vi "2.4 Ghz Cutoff UI.vi"() -> ()   [LabVIEW 2010]
uses:
  Drivers/Telemetry/MICS Parameters Global.vi
  Drivers/Telemetry/MICS_ID Global.vi
  Drivers/Telemetry/MICS_Channel Global.vi
panel:
  in  "Number of \"Open Session\" Retry Attempts (3)":i32=3
  in  "400 MHz MICS Power Setting (0x16)":u8=22 format="%02x"
  in  "Attenuation dB (0)":dbl
  in  "MICS inputs":T1={"address"="COM5", "chan"=2, "ID"=4412} {"ID" format="%04x"; "chan" min=1 max=10 step=1}
  in  "2.45 GHz Wakeup Power Array":i8[](array[ring])=[-29, -4, -2, 0, 2, 4, 6, 8, 10, 12, 14, 16, 18, 20] items=["-29"=-29, "-4"=-4, "-2"=-2, "0"=0, "2"=2, "4"=4, "6"=6, "8"=8, "10"=10, "12"=12, "14"=14, "16"=16, "18"=18, "20"=20, ""=22, ""=24, ""=26, ""=27]
  in  "Samples":i32=10
  in  "stop":bool
  out "error out":errorcluster
  out "Percent Success vs. 2.45 GHz Wakeup Power":T2(graph)
  in  "error in (no error)":errorcluster
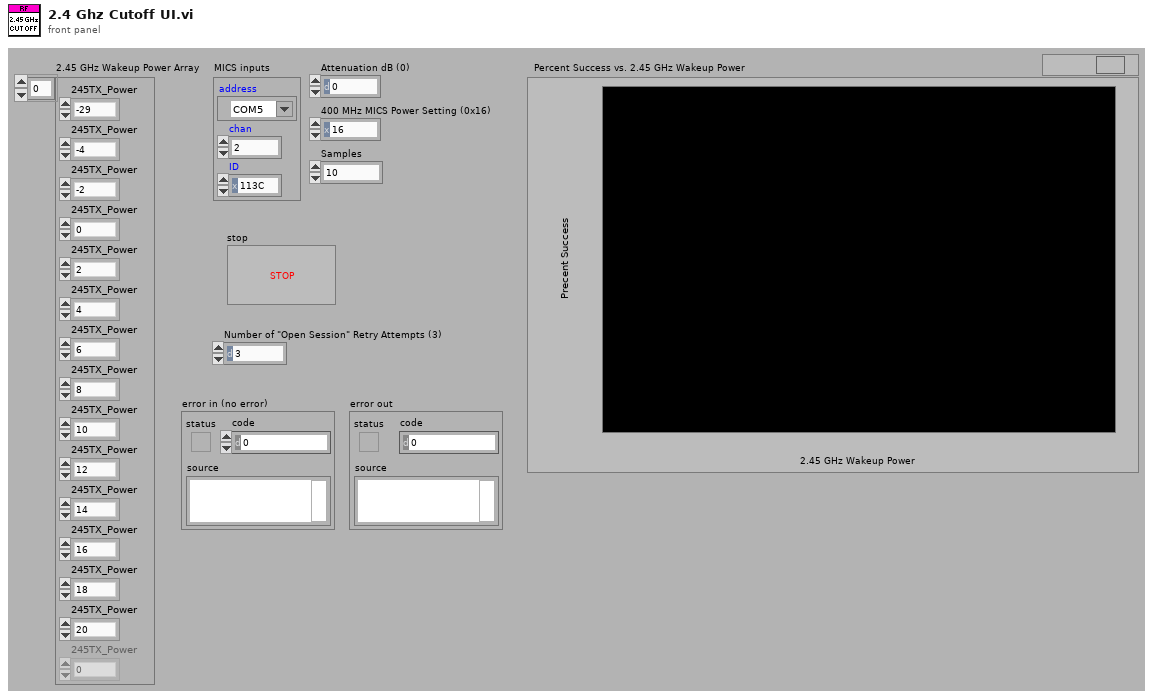
[diagram p1: front panel]
types:
  T1 = cluster{"address":refnum<visa-resource-name>, "chan":u16, "ID":u32}
  T2 = cluster{"245TX_Power":i8, "Percent Successful":dbl}[]
  T3 = cluster{"ConfigFlags":u8, "ImplantID":u32, "CompanyID":u8, "Normal_Comm":cluster{"RF_Channel":u8, "UserData":u8, "TX_Mod":u8, "RX_Mod":u8, "RX_BlockSize":u8, "BlockPerPack":u8, "TX_BlockSize":u8}, "Emerg_Comm":cluster{"RF_Channel":u8, "UserData":u8, "TX_Mod":u8, "RX_Mod":u8, "TX_BlockSize":u8, "BlockPerPack":u8, "RX_BlockSize":u8}, "ImplantRev":u8, "245TX_PowerCal":i8, "245TX_Power":i8, "CCA_RSSI_Thresholds":cluster{"ch0":u16, "ch1":u16, "ch2":u16, "ch3":u16, "ch4":u16, "ch5":u16, "ch6":u16, "ch7":u16, "ch8":u16, "ch9":u16}}
  T4 = cluster{"245TX_Power":i8, "Percent Successful":dbl}
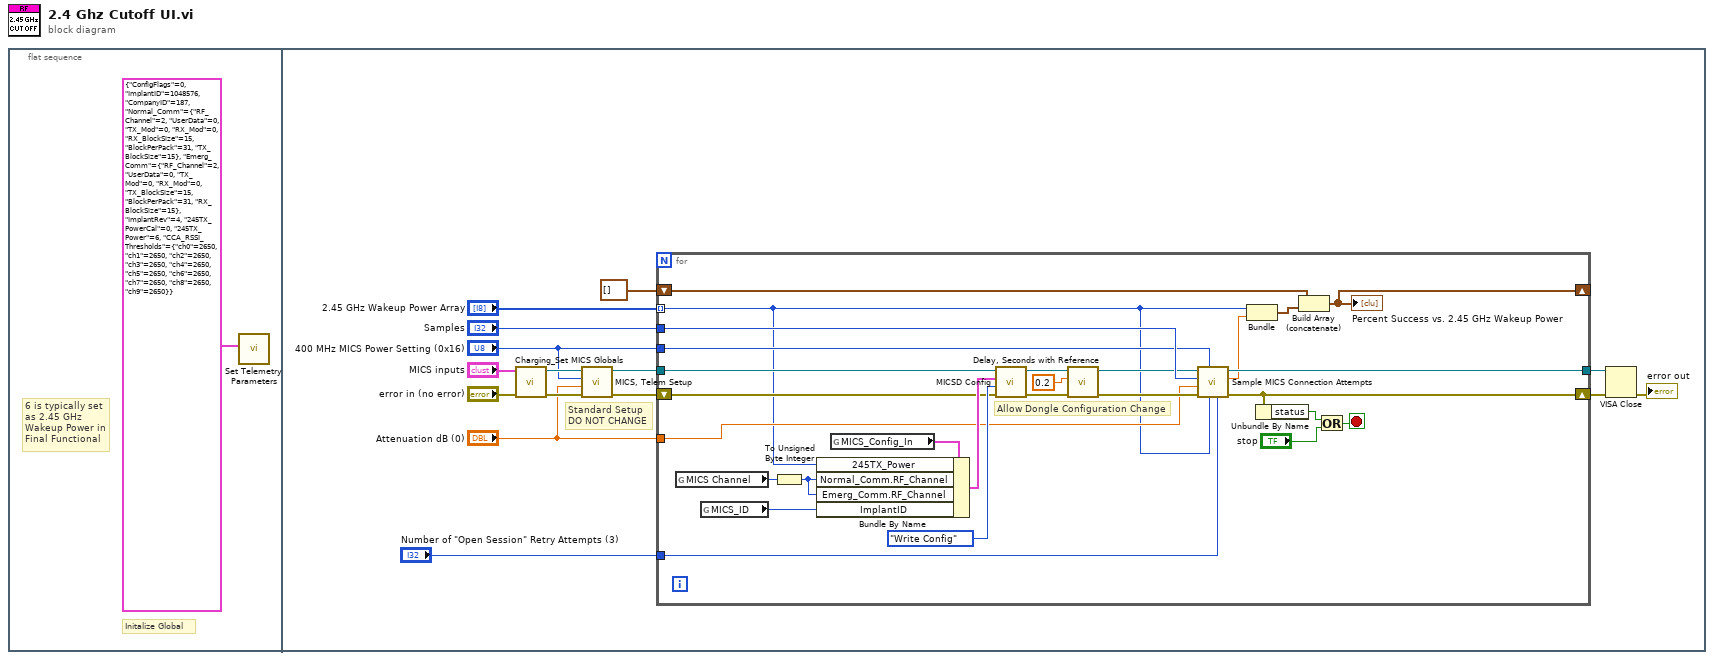
[diagram p0: block diagram]
diagram:
  n1 = flat-sequence {
    frame #0 {
      # "6 is typically set\nas 2.45 GHz\nWakeup Power in\nFinal Functional"
      # "Initalize Global"
      n2 = call "Set Telemetry Parameters.vi"("MICS_Config_In"=T3 {"ConfigFlags"=0, "ImplantID"=1048576, "CompanyID"=187, "Normal_Comm"={"RF_Channel"=2, "UserData"=0, "TX_Mod"=0, "RX_Mod"=0, "RX_BlockSize"=15, "BlockPerPack"=31, "TX_BlockSize"=15}, "Emerg_Comm"={"RF_Channel"=2, "UserData"=0, "TX_Mod"=0, "RX_Mod"=0, "TX_BlockSize"=15, "BlockPerPack"=31, "RX_BlockSize"=15}, "ImplantRev"=4, "245TX_PowerCal"=0, "245TX_Power"=6, "CCA_RSSI_Thresholds"={"ch0"=2650, "ch1"=2650, "ch2"=2650, "ch3"=2650, "ch4"=2650, "ch5"=2650, "ch6"=2650, "ch7"=2650, "ch8"=2650, "ch9"=2650}}) -> ()  [unwired: 11 in]
    }
    frame #1 {
      # "Standard Setup\nDO NOT CHANGE"
      n3 = call "Charging_Set MICS Globals.vi"("error in"="error in (no error)", "MICS inputs"="MICS inputs") -> ("error out"=w13:errorcluster, "address"=w14:refnum<visa-resource-name>)  [unwired: 4 in]
      n4 = call "MICS, Telem Setup.vi"("error in"=w13, "Attenuation dB (0)"="Attenuation dB (0)", "400 MHz MICS Power Setting (0x16)"="400 MHz MICS Power Setting (0x16)", "VISA resource"=w14) -> ("error out"=w6:errorcluster, "VISA resource dup"=w5:refnum<visa-resource-name>)  [unwired: 6 in]
      n5 = for {
        tunnel: w5 -> [w26]
        shift-right: [w42] -> _
        shift-left: cluster{i8, dbl}[] [] ("XY Graph") -> [w43]
        tunnel: [w41] -> w8
        tunnel: "Samples" -> [w35]
        tunnel: "400 MHz MICS Power Setting (0x16)" -> [w34]
        tunnel: "2.45 GHz Wakeup Power Array" -> [w18] mode=indexing
        shift-right: [w40] -> w9
        shift-left: w6 -> [w25]
        tunnel: "Attenuation dB (0)" -> [w19]
        tunnel: "Number of \"Open Session\" Retry Attempts (3)" -> [w17]
        stop <- w38 stop-if-true
        # "Allow Dongle Configuration Change"
        n6 = global read "MICS_Channel Global.vi" "MICS Channel"() -> (w30:u16)
        n7 = global read "MICS_ID Global.vi" "MICS_ID"() -> (w29:u32)
        n8 = To Unsigned Byte Integer(number=w30) -> (unsigned 8bit integer=w28:u8)
        n9 = global read "MICS Parameters Global.vi" "MICS_Config_In"() -> (w31:T3)
        n10 = Bundle By Name(cluster=w31, "245TX_Power"=w18, "Normal_Comm.RF_Channel"=w28, "Emerg_Comm.RF_Channel"=w28, "ImplantID"=w29) -> (w32:T3)
        n11 = call "MICSD Config.vi"("error in (no error)"=w25, "Function"=enum16{"Write Config", "Read Config"}."Write Config", "MICS_Config_In"=w32, "VISA Resource Name"=w26) -> ("error out"=w24:errorcluster, "dup VISA Resource Name"=w22:refnum<visa-resource-name>)  [unwired: 5 in, 1 out]
        n12 = call "Delay, Seconds with Reference.vi"("error in"=w24, "delay"=dbl[unit] 0.2, "VISA resource"=w22) -> ("error out"=w23:errorcluster, "VISA resource dup"=w21:refnum<visa-resource-name>)  [unwired: 3 in, 1 out]
        n13 = call "Sample MICS Connection Attempts.vi"("Number of \"Open Session\" Retry Attempts (3)"=w17, "2.45 GHz Wake-Up Power"=w18, "400 MHz MICS Power Setting"=w34, "error in"=w23, "Attenuation dB"=w19, "Samples (1)"=w35, "MICS Resource Name"=w21) -> ("error out"=w40:errorcluster, "Percent Successful"=w36:dbl, "MICS Resource Name out"=w41:refnum<visa-resource-name>)  [unwired: 1 in, 1 out]
        n14 = Bundle("245TX_Power"=w18, "Percent Successful"=w36) -> (w33:T4)  [unwired: 1 in]
        n15 = Unbundle By Name(w40) -> ("status"=w39:bool)
        n16 = Build Array (concatenate)(w43, w33) -> (w42:T2)
        "Percent Success vs. 2.45 GHz Wakeup Power" <- w42
        n17 = Or(x=w39, y="stop") -> (x .or. y?=w38:bool)
      }
      n18 = VISA Close(VISA resource name=w8, error in (no error)=w9) -> (error out=→"error out":errorcluster)
    }
  }
